vi "SupportAttackerRole_init.vi"(8 "error in (no error)":errorcluster, 10 "roleIndex":u8, 11 "SupportAttackerRole in":refnum<class "SupportAttackerRole.lvclass">) -> (0 "error out":errorcluster, 3 "SupportAttackerRole out":refnum<class "SupportAttackerRole.lvclass">)   [LabVIEW 2023, in "SupportAttackerRole.lvclass"]
uses:
  SupportAttackerRole.lvclass
  C:/Users/ebert/Documents/codes/SSL/repo/SSL_AI/NewSTP/NewRoles/Role_v2_class/Role_v2.lvclass
  NewSTP/Evaluators/SupportAttackerPosition_class/SupportAttackerPosition.lvclass
  C:/Users/ebert/Documents/codes/SSL/repo/SSL_AI/NewSTP/Evaluators/Evaluator_class/Evaluator.lvclass
  PositionTactic_class/PositionTactic.lvclass
  C:/Users/ebert/Documents/codes/SSL/repo/SSL_AI/NewSTP/NewTactics/Tactic_v2_class/Tactic_v2.lvclass
  WaitPassTactic_v2_class/WaitPassTactic_v2.lvclass
  NewSTP/NewRoles/Role_v2_class/Role_v2.lvclass/Role_v2.ctl
  NewSTP/NewRoles/Role_v2_class/Write Tactics.vi
  NewSTP/NewRoles/Role_v2_class/Role_v2.lvclass
  NewSTP/NewTactics/HaltTactic_v2_class/HaltTactic_v2.lvclass
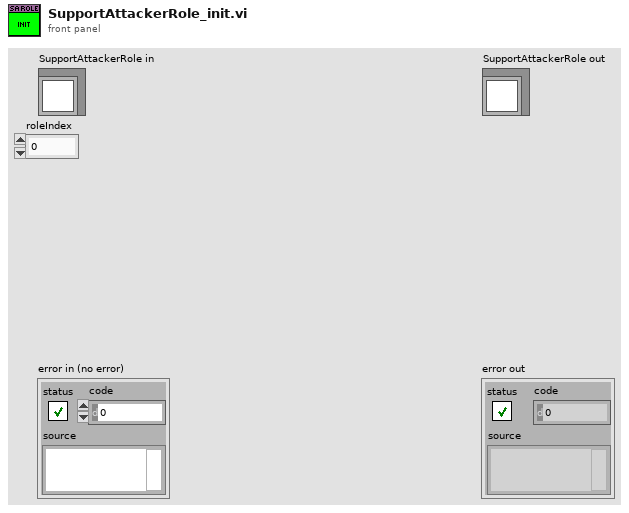
[diagram p1: front panel]
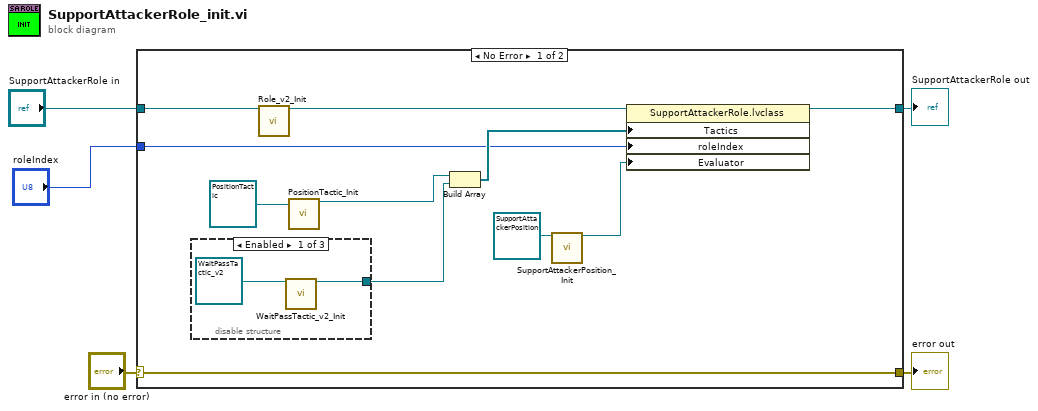
[diagram p0: block diagram]
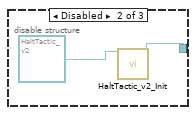
[diagram p2: hidden frame]
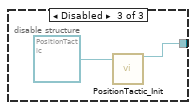
[diagram p3: hidden frame]
diagram:
  n1 = case shown="No Error" "error in (no error)" {
    selector: "error in (no error)" -> [w16 w24]
    tunnel: [w16 w24] -> w4
    tunnel: [w7 w23] -> w2
    tunnel: "SupportAttackerRole in" -> [w14 w23]
    tunnel: "roleIndex" -> [w8 _]
    frame No Error {
      n2 = disable-structure shown="Enabled" {
        disable-tunnel: [w17 w19 w21] -> w9
        frame Enabled {
          n3 = call "WaitPassTactic_v2_Init.vi"("object in"=refnum<class "WaitPassTactic_v2.lvclass"> refnum ("WaitPassTactic_v2")) -> ("object out"=w17:refnum<class "WaitPassTactic_v2.lvclass">)  [unwired: 17 in, 1 out]
        }
        frame Disabled {
          n4 = call "HaltTactic_v2_Init.vi"("object in"=refnum<class "HaltTactic_v2.lvclass"> refnum ("HaltTactic_v2")) -> ("object out"=w19:refnum<class "HaltTactic_v2.lvclass">)  [unwired: 17 in, 1 out]
        }
        frame Disabled {
          n5 = call "PositionTactic_Init.vi"("object in"=refnum<class "PositionTactic.lvclass"> refnum ("PositionTactic")) -> ("object out"=w21:refnum<class "PositionTactic.lvclass">)  [unwired: 17 in, 1 out]
        }
      }
      n6 = call "Role_v2_Init.vi"("object in"=w14) -> ("object out"=w13:refnum<class "SupportAttackerRole.lvclass">)  [unwired: 17 in, 1 out]
      n7 = call "PositionTactic_Init.vi"("object in"=refnum<class "PositionTactic.lvclass"> refnum ("PositionTactic")) -> ("object out"=w11:refnum<class "PositionTactic.lvclass">)  [unwired: 17 in, 1 out]
      n8 = Build Array(w11, w9) -> (w10:refnum<class "Tactic_v2.lvclass">[])
      n9 = call "SupportAttackerPosition_Init.vi"("object in"=refnum<class "SupportAttackerPosition.lvclass"> refnum ("SupportAttackerPosition")) -> ("object out"=w6:refnum<class "SupportAttackerPosition.lvclass">)  [unwired: 17 in, 1 out]
      n10 = property class="SupportAttackerRole.lvclass"(reference=w13, "Tactics"=w10, "roleIndex"=w8, "Evaluator"=w6) -> (reference out=w7:refnum<class "SupportAttackerRole.lvclass">)  [unwired: 1 in, 1 out]
    }
    frame Error {
    }
  }
  "error out" <- w4
  "SupportAttackerRole out" <- w2
